vi "loadRecipeOthersNew.vi"() -> ()   [LabVIEW 2012]
uses:
  <vilib>/Utility/NIReport.llb/NI_report.lvclass
  <vilib>/addons/database/Connection.llb/DB Tools Open Connec (Path).vi
  <vilib>/addons/database/Connection.llb/Conn Execute.vi
  <vilib>/addons/database/Recordset.llb/Rec Destroy - Connection.vi
  <vilib>/Utility/NIReport.llb/Excel/NI_Excel.lvclass
  <vilib>/addons/database/NI_Database_API.lvlib
panel:
  out "output cluster":T1
  out "Numeric":i32
  out "appended path 3":path
  out "error out":errorcluster
  in  "start cell":string="a2"
  out "error out 3":errorcluster
  in  "Cluster":T1
  out "error out 4":errorcluster
  out "data":string[][](array[string])
  out "appended path":path
  in  "path":path=path "O:/Monitor/Recipe/OTHERS"
  out "filenames":string[](array[string])
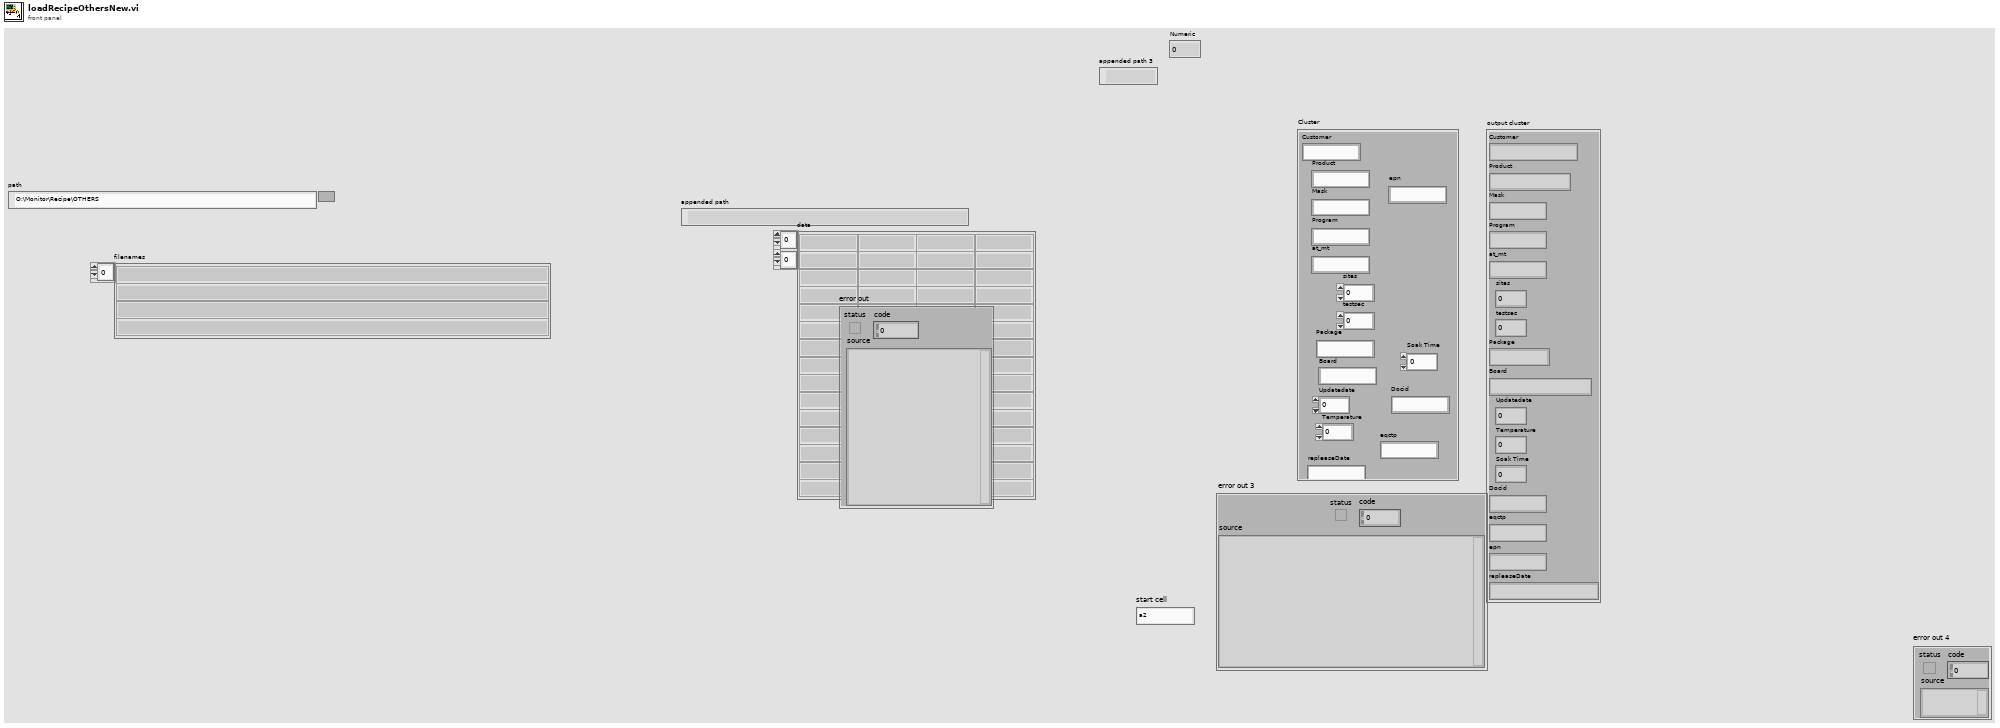
[diagram p1: front panel]
types:
  T1 = cluster{"Customer ":string, "Product":string, "Mask":string, "Program":string, "at_mt":string, "sites ":dbl, "testsec":dbl, "Package":string, "Board ":string, "Updatedate ":dbl, "Temperature":dbl, "Soak Time":dbl, "Docid":string, "eqctp":string, "epn":string, "repleaseDate":string}
  T2 = enum16{"Standard Report", "HTML", "Word", "Excel"}
  T3 = typedef "NI_Database_API.lvlib/Conn ObjectReference.ctl" = refnum<k1>
  T4 = typedef "NI_Database_API.lvlib/Rec ObjectReference.ctl" = refnum<k1>
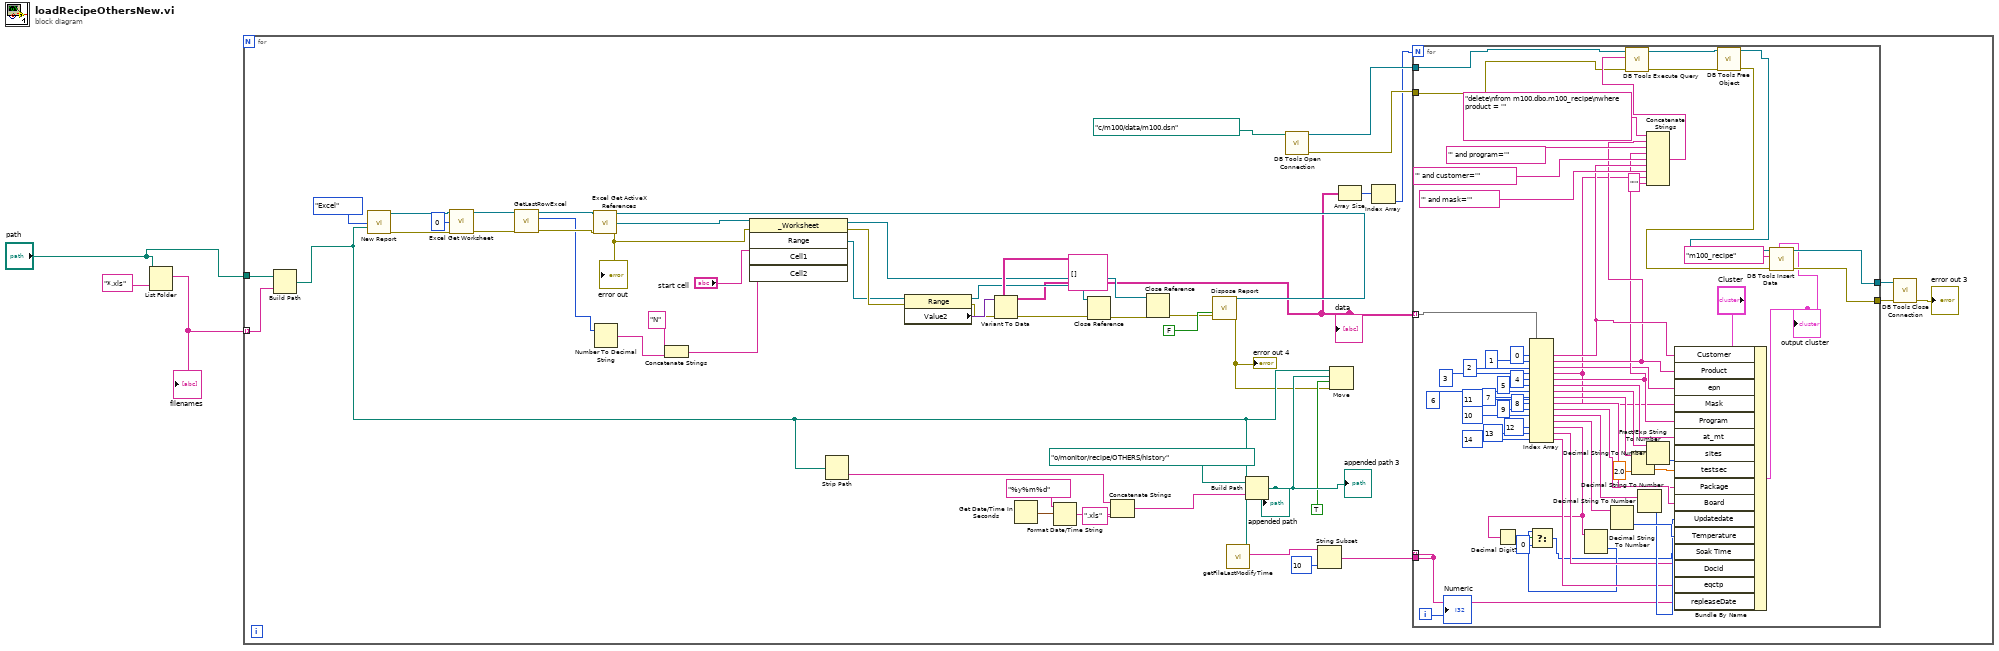
[diagram p0: block diagram]
diagram:
  n1 = List Folder(path="path", pattern="*.xls") -> (filenames=w1:string[])  [unwired: 2 in, 3 out]
  "filenames" <- w1
  n2 = for {
    tunnel: "path" -> [w16]
    tunnel: w1 -> [w15] mode=indexing
    n3 = Build Path(base path=w16, name or relative path=w15) -> (appended path=w7:path)
    n4 = call <vilib>:"New Report.vi"("report type"=T2."Excel", "template (empty)"=w7) -> ("report out"=w54:refnum<class "NI_report.lvclass">, "error out"=w53:errorcluster)  [unwired: 12 in]
    n5 = call <vilib>:"Excel Get Worksheet.vi"("report in"=w54, "worksheet index (0)"=0, "error in (no error)"=w53) -> ("report out"=w35:refnum<class "NI_report.lvclass">, "error out"=w34:errorcluster)  [unwired: 11 in]
    n6 = call "GetLastRowExcel.vi"("error in (no error)"=w34, "report in"=w35) -> ("error out"=w32:errorcluster, "row"=w31:i32, "report out"=w33:refnum<class "NI_report.lvclass">)  [unwired: 7 in]
    n7 = call <vilib>:"Excel Get ActiveX References.vi"("report in"=w33, "error in (no error)"=w32) -> ("report out"=w25:refnum<class "NI_report.lvclass">, "Excel._Worksheet"=w50:refnum<k7>, "error out"=w36:errorcluster)  [unwired: 7 in, 4 out]
    "error out" <- w36
    n8 = Number To Decimal String(number=w31) -> (decimal integer string=w29:string)  [unwired: 1 in]
    n9 = Concatenate Strings("N" ("string"), w29) -> (w28:string)
    n10 = invoke class="_Worksheet" method="Range"(reference=w50, error in=w36, "Cell1"="start cell", "Cell2"=w28) -> (reference out=w42:refnum<k7>, error out=w47:errorcluster, "Range"=w46:refnum<k7>)  [unwired: 1 in, 2 out]
    n11 = Strip Path(path=w7) -> (name=w17:string)  [unwired: 1 out]
    n12 = property class="Range"(reference=w46, error in=w47) -> (reference out=w43:refnum<k7>, error out=w48:errorcluster, "Value2"=w49:variant)
    n13 = Variant To Data(error in=w48, type=string[][] [], Variant=w49) -> (data=w13:string[][], error out=w44:errorcluster)
    "data" <- w13
    n14 = Get Date/Time In Seconds() -> (seconds since 1Jan1904=w22:timestamp)
    n15 = Format Date/Time String(time format string (%c)="%y%m%d", seconds (now)=w22) -> (date/time string=w20:string)  [unwired: 1 in]
    n16 = Close Reference(reference=w43, error in (no error)=w44) -> (error out=w41:errorcluster)
    n17 = Concatenate Strings(w17, w20, ".xls" ("string")) -> (w23:string)
    n18 = Close Reference(reference=w42, error in (no error)=w41) -> (error out=w26:errorcluster)
    n19 = call-dynamic "Dispose Report.vi"("report in"=w25, "save changes? (F)"=FALSE, "error in (no error)"=w26) -> ("error out"=w4:errorcluster)  [unwired: 12 in]
    "error out 4" <- w4
    n20 = call "getFileLastModifyTime.vi"("path"=w7) -> ("date/time string"=w10:string)  [unwired: 10 in]
    n21 = Build Path(base path=path "o:/monitor/recipe/OTHERS/history", name or relative path=w23) -> (appended path=w6:path)
    "appended path" <- w6
    "appended path 3" <- w6
    n22 = call-poly <vilib>:"DB Tools Open Connection.vi"("connection information"=path "c:/m100/data/m100.dsn") -> ("error out"=w18:errorcluster, "connection reference"=w14:T3)  [unwired: 7 in]
    n23 = String Subset(string=w10, length (rest)=10 ("length (rest)")) -> (substring=w9:string)  [unwired: 1 in]
    n24 = Move(source path=w7, error in=w4, 9:TRUE, 10:w6) -> ()  [unwired: 1 in, 3 out]
    n25 = Array Size(array=w13) -> (size(s)=w12:i32[])
    n26 = Index Array(array=w12) -> (element=w11:i32)  [unwired: 1 in]
    n27 = for {
      N: w11 -> [_]
      tunnel: w18 -> [w100]
      tunnel: [w114] -> w38
      tunnel: [w113] -> w37
      tunnel: w13 -> [w112] mode=indexing
      tunnel: w14 -> [w101]
      tunnel: [w58] -> _ mode=indexing
      tunnel: w9 -> [w58]
      i -> [w79]
      n28 = Index Array(array=w112, index #1=0 ("index"), index #2=1 ("index"), index #3=2 ("index"), index #4=3 ("index"), index #5=4 ("index"), index #6=5 ("index"), index #7=6 ("index"), index #8=7 ("index"), index #9=8 ("index"), index #10=9 ("index"), index #11=10 ("index"), index #12=11 ("index"), index #13=12 ("index"), index #14=13 ("index"), index #15=14 ("index")) -> (element #1=w92:string, element #2=w91:string, element #3=w80:string, element #4=w57:string, element #5=w81:string, element #6=w82:string, element #7=w83:string, element #8=w84:string, element #9=w85:string, element #10=w86:string, element #11=w87:string, element #12=w88:string, element #13=w78:string, element #14=w89:string, element #15=w90:string)
      n29 = Decimal Digit?(1:w78) -> (0:w77:bool)
      n30 = Decimal String To Number(string=w78) -> (number=w76:i32)  [unwired: 2 in, 1 out]
      n31 = Select(t=w76, s=w77, f=0) -> (s? t:f=w74:i32)
      n32 = Decimal String To Number(string=w88) -> (number=w109:i32)  [unwired: 2 in, 1 out]
      n33 = Fract/Exp String To Number(string=w84, default (0 dbl)=2.0 ("default (0 DBL)")) -> (number=w107:dbl)  [unwired: 2 in, 1 out]
      n34 = Decimal String To Number(string=w87) -> (number=w108:i32)  [unwired: 2 in, 1 out]
      n35 = Concatenate Strings("delete\nfrom m100.dbo.m100_recipe\nwhere product = '" ("string"), w91, "' and program='" ("string"), w81, "' and customer='" ("string"), w92, "' and mask='" ("string"), w57, "'" ("string")) -> (w102:string)
      n36 = call-poly <vilib>:"DB Tools Execute Query.vi"("error in (no error)"=w100, "SQL query"=w102, "connection reference"=w101) -> ("error out"=w94:errorcluster, "recordset reference"=w95:T4)  [unwired: 5 in]
      n37 = Decimal String To Number(string=w83) -> (number=w106:i32)  [unwired: 2 in, 1 out]
      n38 = Bundle By Name(cluster="Cluster", "Customer"=w92, "Product"=w91, "epn"=w80, "Mask"=w57, "Program"=w81, "at_mt"=w82, "sites"=w106, "testsec"=w107, "Package"=w85, "Board"=w86, "Updatedate"=w108, "Temperature"=w109, "Soak Time"=w74, "Docid"=w89, "eqctp"=w90, "repleaseDate"=w58) -> (w110:T1)
      "output cluster" <- w110
      n39 = call-poly <vilib>:"DB Tools Free Object.vi"("error in (no error)"=w94, "recordset reference"=w95) -> ("error out"=w98:errorcluster, "connection reference"=w99:T3)  [unwired: 8 in]
      n40 = call <vilib>:"DB Tools Insert Data.vi"("data"=w110, "error in (no error)"=w98, "table"="m100_recipe", "connection reference"=w99) -> ("error out"=w113:errorcluster, "connection reference out"=w114:T3)  [unwired: 6 in]
      "Numeric" <- w79
    }
    n41 = call <vilib>:"DB Tools Close Connection.vi"("error in (no error)"=w37, "connection reference"=w38) -> ("error out"=→"error out 3":errorcluster)  [unwired: 5 in]
  }
